vi "sin_func_glob_var.vi"(8 "error constant":errorcluster, 11 "dx":dbl) -> (0 "error constant 2":errorcluster, 3 "sin x":dbl)   [LabVIEW 2022 SP3]
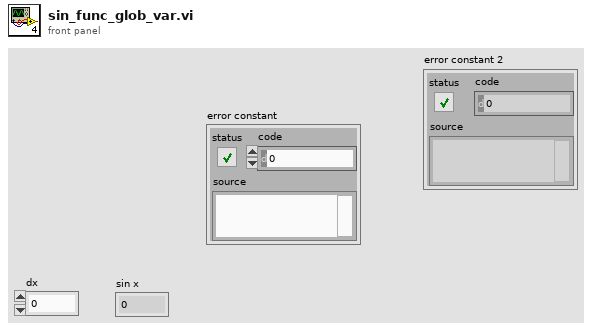
[diagram p1: front panel]
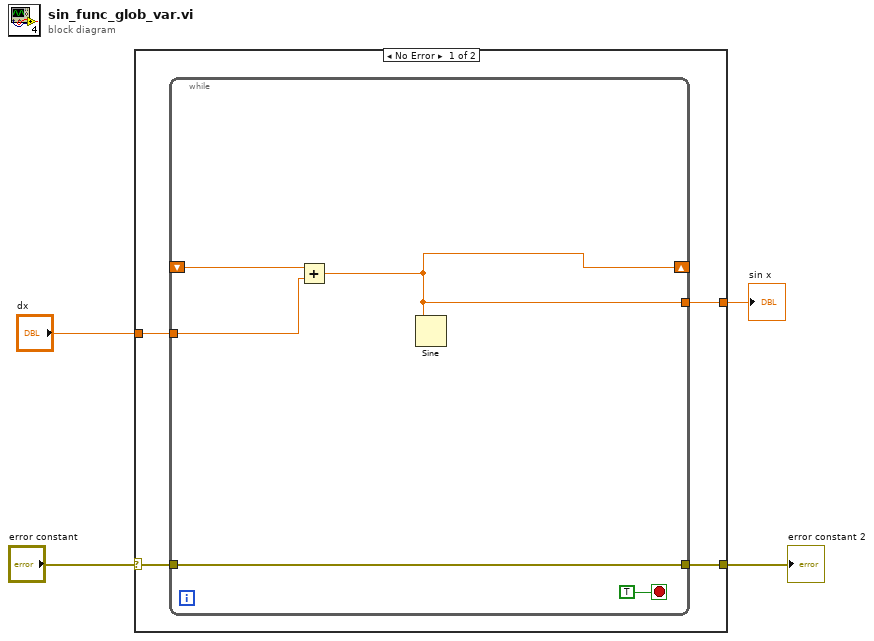
[diagram p0: block diagram]
diagram:
  n1 = case shown="No Error" "error constant" {
    selector: "error constant" -> [w7 w14]
    tunnel: "dx" -> [w8 _]
    tunnel: [w6 w14] -> w2
    tunnel: [w5 _] -> w1
    frame No Error {
      n2 = while {
        shift-right: [w9] -> _
        shift-left: _ -> [w12]
        tunnel: w8 -> [w11]
        tunnel: [w10] -> w6
        tunnel: w7 -> [w10]
        tunnel: [w9] -> w5
        stop <- TRUE stop-if-true
        n3 = Add(x=w12, y=w11) -> (x+y=w9:dbl)
        n4 = Sine(x=w9) -> ()  [unwired: 1 out]
      }
    }
    frame Error {
    }
  }
  "error constant 2" <- w2
  "sin x" <- w1
